vi "StringToChannelsArray.vi"(8 "error in (no error)":errorcluster, 10 "String":string) -> (0 "error out":errorcluster, 1 "String Array":string[](array[string]), 2 "Channels Array":T1[](array[typedef]))   [LabVIEW 2016, in "pickering.lvclass"]
uses:
  pickering.lvclass
  Typedefs/Channel-Cluster.ctl
  Typedefs/ChannelX-ComboBox.ctl
  Typedefs/ChannelY-ComboBox.ctl
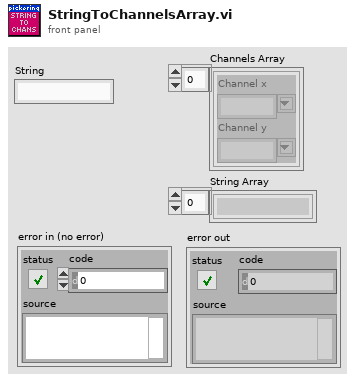
[diagram p1: front panel]
types:
  T1 = typedef "pickering.lvclass/Channel-Cluster.ctl" = cluster{"Channel x":T2, "Channel y":T3}
  T2 = typedef "pickering.lvclass/ChannelX-ComboBox.ctl" = string
  T3 = typedef "pickering.lvclass/ChannelY-ComboBox.ctl" = string
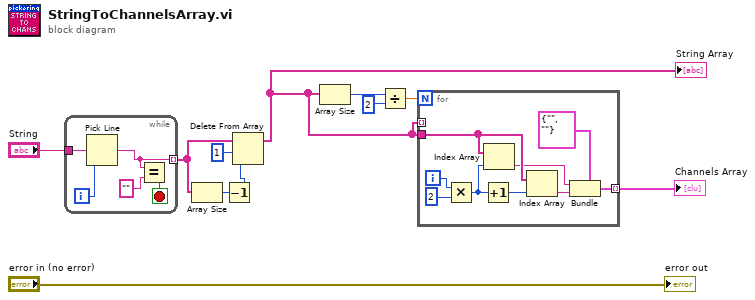
[diagram p0: block diagram]
diagram:
  n1 = while {
    tunnel: "String" -> [w16]
    tunnel: [w14] -> w6 mode=indexing
    i -> [w15]
    stop <- w12 stop-if-true
    n2 = Pick Line(multi-line string=w16, line index=w15) -> (output string=w14:string)  [unwired: 1 in]
    n3 = Equal?(x=w14, y="" ("output string")) -> (x = y?=w12:bool)
  }
  n4 = Array Size(array=w6) -> (size(s)=w3:i32)
  n5 = Decrement(x=w3) -> (x-1=w4:i32)
  n6 = Delete From Array(array=w6, length=1, index=w4) -> (array with subset deleted=w10:string[])  [unwired: 1 out]
  "String Array" <- w10
  n7 = Array Size(array=w10) -> (size(s)=w7:i32)
  n8 = Divide(x=w7, y=2) -> (x/y=w9:dbl)
  n9 = for {
    N: w9 -> [_]
    tunnel: w10 -> [w25]
    tunnel: w10 -> [_] mode=indexing
    tunnel: [w21] -> w11 mode=indexing
    i -> [w20]
    n10 = Multiply(x=w20, y=2) -> (x*y=w18:i32)
    n11 = Increment(x=w18) -> (x+1=w24:i32)
    n12 = Index Array(array=w25, index=w18) -> (element=w23:string)
    n13 = Index Array(array=w25, index=w24) -> (element=w22:string)
    n14 = Bundle(cluster=T1 {"Channel x"="", "Channel y"=""} ("Cluster"), "Channel x"=w23, "Channel y"=w22) -> (w21:T1)
  }
  "Channels Array" <- w11
  "error out" <- "error in (no error)"
